vi "Teleop.vi"(10 "Match Info":T1={"Autonomous Elapsed Seconds"=0.0, "TeleOp Elapsed Seconds"=0.0, "Disabled Elapsed Seconds"=0.0, "Visited Autonomous"=FALSE, "Visited TeleOp"=FALSE, "Visited Disabled"=FALSE, "Autonomous Settings"={"Autonomous Style"=enum."Independent", "VI Refnum"=refnum}}, 11 "Call Context":T2) -> ()   [LabVIEW 2017]
doc: "This VI is called for each TeleOp packet received from the DS where the robot is not disabled. It is often used to read from the joysticks and update I/O or to update setpoints for timed control loops. It should complete and return within 20 milliseconds or it may miss DS packets."
uses:
  <vilib>/Rock Robotics/WPI/DriverStation/WPI_DriverStationDerivedRobotMode.ctl
  <vilib>/Rock Robotics/WPI/DriverStation/WPI_DriverStationMatch Info.ctl
  C:/Users/Public/Documents/Cross The Road Electronics/Phoenix-LabVIEW/Motor Controller/Controls/CTRE_Phoenix_MotorControl_ControlMode.ctl
  <vilib>/Rock Robotics/WPI/Utilities/WPI_GetSetVariantRefNum.vi
  <vilib>/Rock Robotics/Network Tables/NT Write Boolean Array.vi
  <vilib>/Rock Robotics/Network Tables/NT Write Numeric Array.vi
  C:/Users/Public/Documents/Cross The Road Electronics/Phoenix-LabVIEW/Motor Controller/Get/CTRE_Phoenix_MotorController_GetVoltage.vi
  C:/Users/Public/Documents/Cross The Road Electronics/Phoenix-LabVIEW/Motor Controller/Get/CTRE_Phoenix_MotorController_GetOutputCurrent_Enhanced.vi
panel:
  in  "I Zone":dbl
  in  "F":dbl
  in  "D":dbl
  in  "I":dbl
  in  "P":dbl
  out "Requested Current Amps":dbl
  out "Applied Throttle":dbl
  out "Current Draw Amps":dbl
  # "When Button1 is released, y-axis controls the Talon SRX drive directly.\nWhen Button1 is held, y-axis closed-loops the target-current-draw.\n\nWhen Button2 is held, the Closed-Loop gain parameters are sent to Talon.\n\nCalcFgain = 100% X 1023 / CurrentMeasMilliAmps , assuming measurement was at 100% motor output.\n\nFor example, if the CurrentDraw indicator reads 30.125 A at 75.56% throttle , the calculated Fgain is....\nCalcFgain = 0.7556 X 1023 / 30125\nCalcFgain = 0.02566"
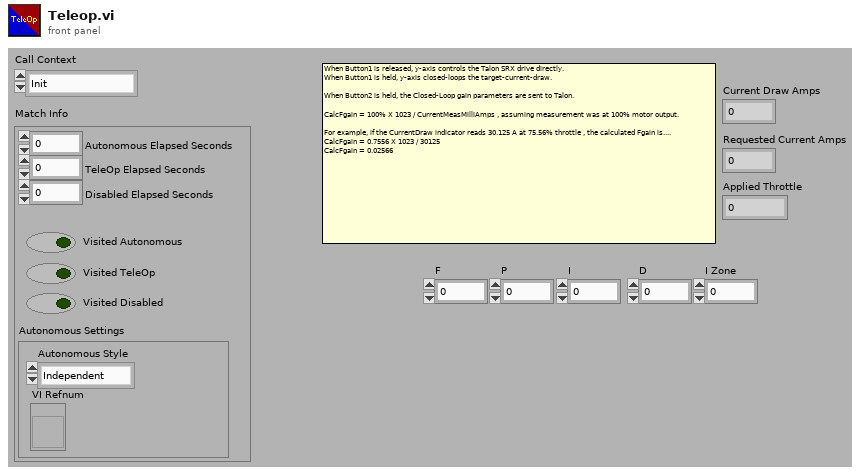
[diagram p1: front panel]
types:
  T1 = typedef "WPI_DriverStationMatch Info.ctl" = cluster{"Autonomous Elapsed Seconds":dbl, "TeleOp Elapsed Seconds":dbl, "Disabled Elapsed Seconds":dbl, "Visited Autonomous":bool, "Visited TeleOp":bool, "Visited Disabled":bool, "Autonomous Settings":cluster{"Autonomous Style":enum16{"Iterative", "Independent"}, "VI Refnum":refnum<vi>}}
  T2 = typedef "WPI_DriverStationDerivedRobotMode.ctl" = enum16{"Init", "Execute", "Stop"}
  T3 = typedef "WPI_JoystickDevRef.ctl" = cluster{"Device":T4}
  T4 = typedef "WPI_JoystickDeviceEnum.ctl" = enum16{"USB 0", "USB 1", "USB 2", "USB 3", "USB 4", "USB 5"}
  T5 = typedef "WPI_MotorControlDeviceRef.ctl" = cluster{"DeviceStatus":errorcluster, "Type":T6, "PWM":cluster{"PWM Channel":T7, "DeadBand":T8}, "CAN":cluster{"Device Number":u8, "SetOutput VI Ref":variant, "GetOutput VI Ref":variant, "Enable VI Ref":variant, "Disable VI Ref":variant, "Data":variant}, "Invert":bool, "DIO PWM":cluster{"PWM \"Enable\" Channel":T7, "DIOChannel":T9, "PWM Rate":dbl}}
  T6 = typedef "WPI_MotorControlType.ctl" = enum16{"PWM", "CAN", "DIO PWM"}
  T7 = typedef "FPGA_DIOPWMChannel.ctl" = enum8{"PWM 0", "PWM 1", "PWM 2", "PWM 3", "PWM 4", "PWM 5", "PWM 6", "PWM 7", "PWM 8", "PWM 9", "PWM MXP 0", "PWM MXP 1", "PWM MXP 2", "PWM MXP 3", "PWM MXP 4", "PWM MXP 5", "PWM MXP 6", "PWM MXP 7", "PWM MXP 8", "PWM MXP 9", "Invalid"}
  T8 = typedef "WPI_PWMDeadband.ctl" = cluster{"Name":string, "maxPositivePwm":i32, "minPositivePwm":i32, "centerPwm":i32, "maxNegativePwm":i32, "minNegativePwm":i32, "angularRange":u16}
  T9 = typedef "FPGA_DIOChannel.ctl" = enum8{"DIO 0", "DIO 1", "DIO 2", "DIO 3", "DIO 4", "DIO 5", "DIO 6", "DIO 7", "DIO 8", "DIO 9", "DIO MXP 0", "DIO MXP 1", "DIO MXP 2", "DIO MXP 3", "DIO MXP 4", "DIO MXP 5", "DIO MXP 6", "DIO MXP 7", "DIO MXP 8", "DIO MXP 9", "DIO MXP 10", "DIO MXP 11", "DIO MXP 12", "DIO MXP 13", "DIO MXP 14", "DIO MXP 15", "SPI Port CS1", "SPI Port CS2", "SPI Port CS3", "SPI Port MISO", "SPI Port MOSI", "Invalid"}
  T10 = typedef "CTRE_Phoenix_MotorControl_ControlMode.ctl" = u16
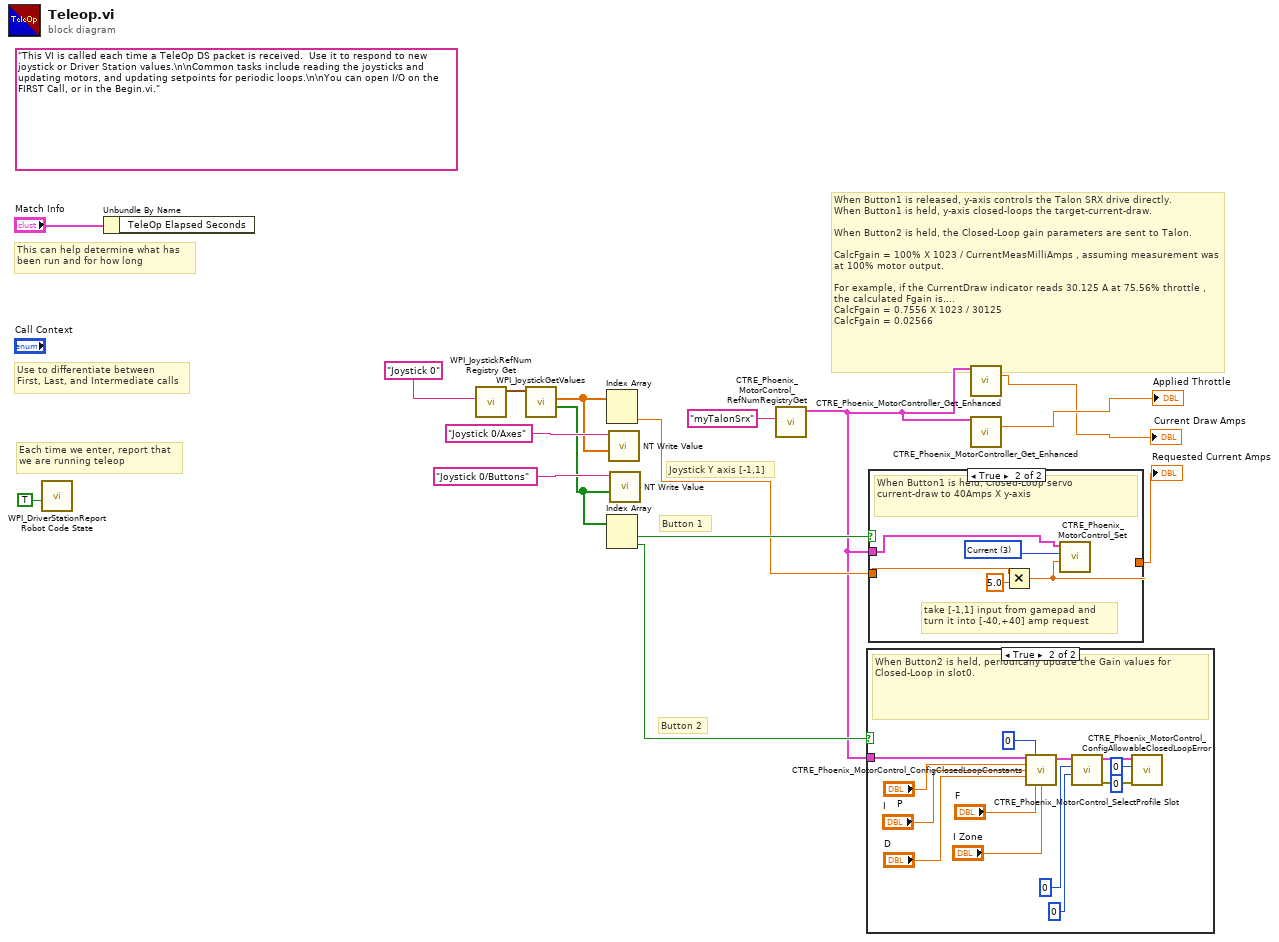
[diagram p0: block diagram]
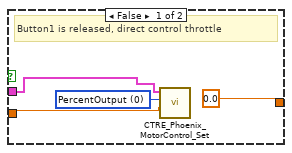
[diagram p3: hidden frame]
diagram:
  (unwired) "This VI is called each time a TeleOp DS packet is received.  Use it to respond to new joystick or Driver Station values.\n\nCommon tasks include reading the joysticks and updating motors, and updating setpoints for periodic loops.\n\nYou can open I/O on the FIRST Call, or in the Begin.vi."
  # "Button 2"
  # "When Button1 is released, y-axis controls the Talon SRX drive directly.\nWhen Button1 is held, y-axis closed-loops the target-current-draw.\n\nWhen Button2 is held, the Closed-Loop gain parameters are sent to Talon.\n\nCalcFgain = 100% X 1023 / CurrentMeasMilliAmps , assuming measurement was at 100% motor output.\n\nFor example, if the CurrentDraw indicator reads 30.125 A at 75.56% throttle , the calculated Fgain is....\nCalcFgain = 0.7556 X 1023 / 30125\nCalcFgain = 0.02566"
  # "Button 1"
  # "Joystick Y axis [-1,1]"
  # "Each time we enter, report that\nwe are running teleop"
  # "Use to differentiate between\nFirst, Last, and Intermediate calls"
  # "This can help determine what has\nbeen run and for how long"
  n1 = call <vilib>:"WPI_DriverStationReport Robot Code State.vi"("TeleOp"=TRUE ("Autonomous")) -> ()  [unwired: 10 in, 1 out]
  n2 = Unbundle By Name("Match Info") -> ()  [unwired: 1 out]
  n3 = call <vilib>:"WPI_JoystickRefNum Registry Get.vi"("refnum name"="Joystick 0") -> ("JoystickDevRef"=w14:T3)  [unwired: 1 in, 9 out]
  n4 = call <vilib>:"WPI_JoystickGetValues.vi"("JoystickDevRef"=w14) -> ("Buttons"=w8:bool[], "Axes"=w10:dbl[])  [unwired: 6 in, 3 out]
  n5 = Index Array(array=w10) -> (element #2=w5:dbl)  [unwired: 2 in, 1 out]
  n6 = Index Array(array=w8) -> (element #1=w6:bool, element #2=w4:bool)  [unwired: 2 in]
  n7 = call-poly <vilib>:"NT Write Value.vi"("Numeric Array"=w10, "Name"="Joystick 0/Axes") -> ()  [unwired: 9 in, 1 out]
  n8 = call-poly <vilib>:"NT Write Value.vi"("Boolean Array"=w8, "Name"="Joystick 0/Buttons") -> ()  [unwired: 9 in, 1 out]
  n9 = call "CTRE_Phoenix_MotorControl_RefNumRegistryGet.vi"("refnum name"="myTalonSrx") -> ("PhoenixMotorControlDevRef"=w1:T5)  [unwired: 9 in, 1 out]
  n10 = case shown="True" w4 {
    tunnel: w1 -> [_ w25]
    frame False {
    }
    frame True {
      # "When Button2 is held, periodically update the Gain values for Closed-Loop in slot0."
      n11 = call "CTRE_Phoenix_MotorControl_ConfigClosedLoopConstants.vi"("PhoenixMotorControlDevRef"=w25, "slotIdx"=0 ("Parameter Slot"), "P"="P", "I"="I", "D"="D", "F"="F", "I Zone"="I Zone") -> ("PhoenixMotorControlDevRef"=w23:T5)  [unwired: 7 in, 1 out]
      n12 = call "CTRE_Phoenix_MotorControl_SelectProfile Slot.vi"("pidLoopIdx"=0, "slotIdx"=0, "PhoenixMotorControlDevRef"=w23) -> ("error out"=w20:errorcluster, "PhoenixMotorControlDevRef"=w19:T5)  [unwired: 7 in]
      n13 = call "CTRE_Phoenix_MotorControl_ConfigAllowableClosedLoopError.vi"("error in (no error)"=w20, "slotIdx"=u32 0, "allowableClosedLoopError"=0, "PhoenixMotorControlDevRef"=w19) -> ()  [unwired: 6 in, 2 out]
    }
  }
  n14 = case shown="True" w6 {
    tunnel: w5 -> [w32 w39]
    tunnel: w1 -> [w33 w37]
    tunnel: [0.0 w36] -> w7
    frame False {
      w31 = T10 0 items=["PercentOutput"=0, "Position"=1, "Velocity"=2, "Current"=3, "Follower"=5, "MotionProfile"=6, "MotionMagic"=7, "MotionMagicArc"=8, "TimedPercentOutput"=9, "Disabled"=15] ("Control Mode")
      # "Button1 is released, direct control throttle"
      n15 = call "CTRE_Phoenix_MotorControl_Set.vi"("Output"=w32, "Control Mode"=w31, "PhoenixMotorControlDevRef"=w33) -> ()  [unwired: 7 in, 2 out]
    }
    frame True {
      w35 = T10 3 items=["PercentOutput"=0, "Position"=1, "Velocity"=2, "Current"=3, "Follower"=5, "MotionProfile"=6, "MotionMagic"=7, "MotionMagicArc"=8, "TimedPercentOutput"=9, "Disabled"=15] ("Control Mode")
      # "take [-1,1] input from gamepad and \nturn it into [-40,+40] amp request"
      # "When Button1 is held, Closed-Loop servo \ncurrent-draw to 40Amps X y-axis"
      n16 = Multiply(x=w39, y=5.0) -> (x*y=w36:dbl)
      n17 = call "CTRE_Phoenix_MotorControl_Set.vi"("Output"=w36, "Control Mode"=w35, "PhoenixMotorControlDevRef"=w37) -> ()  [unwired: 7 in, 2 out]
    }
  }
  "Requested Current Amps" <- w7
  n18 = call-poly "CTRE_Phoenix_MotorController_Get_Enhanced.vi"("PhoenixMotorControlDevRef"=w1) -> ("Output Current"=→"Current Draw Amps":dbl)  [unwired: 12 in, 2 out]
  n19 = call-poly "CTRE_Phoenix_MotorController_Get_Enhanced.vi"("PhoenixMotorControlDevRef"=w1) -> ("Percent Output"=→"Applied Throttle":dbl)  [unwired: 10 in, 4 out]
